vi "Try Parse.vi"(0 "Vector Path in":refnum<class "Vector 26GHz Path.lvclass">, 5 "Config Row":string[](array[string]), 11 "error in (no error)":errorcluster) -> (4 "Vector Path out":refnum<class "Vector 26GHz Path.lvclass">, 6 "Is of type?":bool, 15 "error out":errorcluster)   [LabVIEW 2023, in "RFFixtureCharact.RMM.lvlib" / "Vector 26GHz Path.lvclass"]
uses:
  Vector 26GHz Path.lvclass
  Vector 26GHz Path.lvclass/Vector 26GHz Path.ctl
  Common/RFCalAndFixtureCharact.Common.lvlib
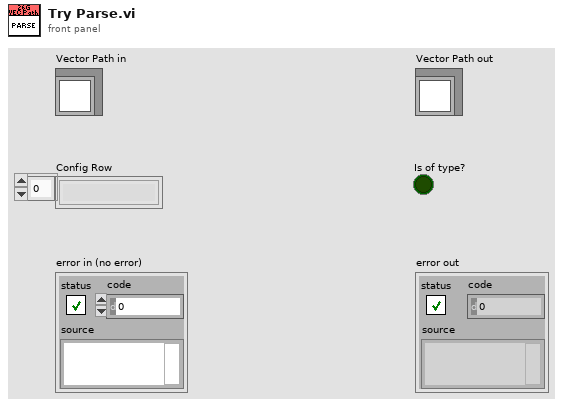
[diagram p1: front panel]
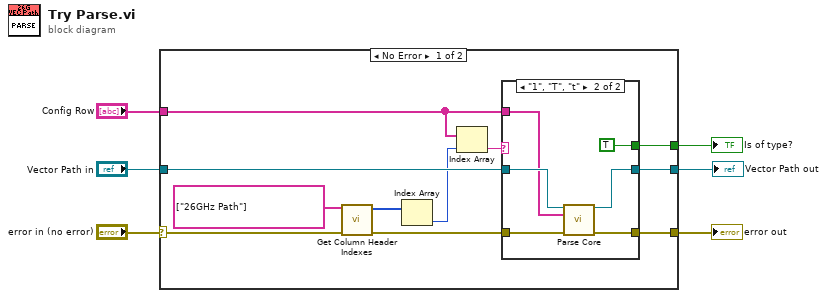
[diagram p0: block diagram]
diagram:
  n1 = case shown="No Error" "error in (no error)" {
    selector: "error in (no error)" -> [w16 w27]
    tunnel: [w10 w27] -> w1
    tunnel: [w17 _] -> w3
    tunnel: [w11 w26] -> w2
    tunnel: "Config Row" -> [w14 _]
    tunnel: "Vector Path in" -> [w15 w26]
    frame No Error {
      n2 = call "Get Column Header Indexes.vi"("Column Header Names"=string[] ["26GHz Path"], "error in"=w16) -> ("Column Header Indices"=w8:i32[], "error out"=w9:errorcluster)  [unwired: 11 in, 1 out]
      n3 = Index Array(array=w8) -> (element=w7:i32)  [unwired: 1 in]
      n4 = Index Array(array=w14, index=w7) -> (element=w13:string)
      n5 = case shown="\"1\", \"T\", \"t\"" w13 {
        tunnel: [w18 w21] -> w10
        tunnel: [_ TRUE ("Is of type?")] -> w17
        tunnel: [w19 w23] -> w11
        tunnel: w9 -> [w18 w22]
        tunnel: w15 -> [w19 w24]
        tunnel: w14 -> [_ w20]
        frame Default {
        }
        frame "1", "T", "t" {
          n6 = call-dynamic "Parse Core.vi"("Vector Path in"=w24, "Config Row"=w20, "error in (no error)"=w22) -> ("Vector Path out"=w23:refnum<class "Vector 26GHz Path.lvclass">, "error out"=w21:errorcluster)  [unwired: 11 in]
        }
      }
    }
    frame Error {
    }
  }
  "error out" <- w1
  "Vector Path out" <- w2
  "Is of type?" <- w3
